vi "MeasAction.vi"(8 "error in (no error)":errorcluster caption="entrée d'erreur (pas d'erreur)", 9 "CurvePointIndex":i32, 10 "AllPointIndex":i32, 11 "InstrClassIn":refnum<class "SymphonyCCD.lvclass"> caption="DNL_LabVIEW Object in") -> (0 "error out":errorcluster caption="sortie d'erreur", 2 "MeasDatOut":dbl[](array[numeric]), 3 "InstrClassOut":refnum<class "SymphonyCCD.lvclass"> caption="DNL_LabVIEW Object out")   [LabVIEW 2019, in "SymphonyCCD.lvclass"]
uses:
  SymphonyCCD.lvclass
  SymphonyCCD.lvclass/SymphonyCCD.ctl
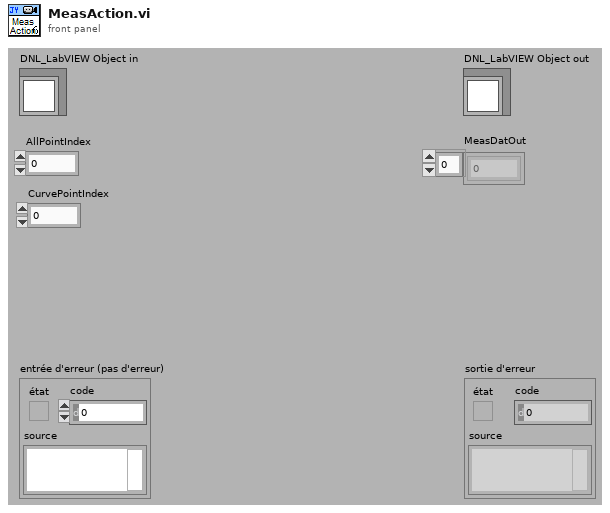
[diagram p1: front panel]
types:
  T1 = typedef "SymphonyCCD.lvclass/SymphonyCCD_Func.ctl" = enum16{"AcqImageSim (Counts)", "AcqImage (Counts)"}
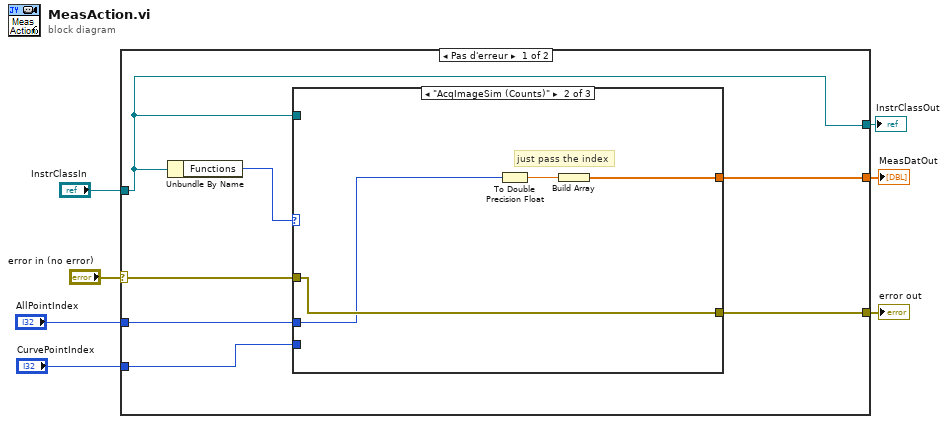
[diagram p0: block diagram]
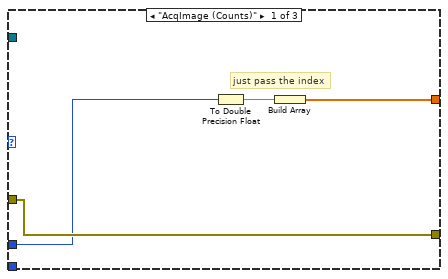
[diagram p2: hidden frame]
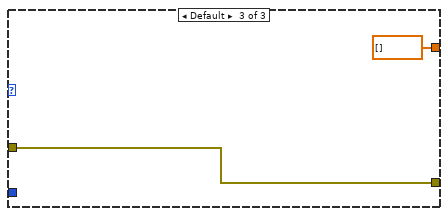
[diagram p3: hidden frame]
diagram:
  n1 = case shown="Pas d'erreur" "error in (no error)" {
    selector: "error in (no error)" -> [w10 w25]
    tunnel: "InstrClassIn" -> [w8 w26]
    tunnel: [w8 w26] -> w5
    tunnel: "AllPointIndex" -> [w14 _]
    tunnel: [w13 w25] -> w3
    tunnel: [w12 _] -> w2
    tunnel: "CurvePointIndex" -> [w9 _]
    frame No Error {
      n2 = Unbundle By Name(w8) -> ("Functions"=w11:T1)
      n3 = case shown="\"AcqImageSim (Counts)\"" w11 {
        tunnel: w14 -> [w15 w19 _]
        tunnel: [w18 w22 w23] -> w13
        tunnel: [w16 w20 dbl[] [] ("Outputs")] -> w12
        tunnel: w10 -> [w18 w22 w23]
        tunnel: w9 -> [_ _ _]
        tunnel: w8 -> [_ _ _]
        frame "AcqImage (Counts)" {
          # "just pass the index"
          n4 = To Double Precision Float(number=w15) -> (double precision float=w17:dbl)
          n5 = Build Array(w17) -> (w16:dbl[])
        }
        frame "AcqImageSim (Counts)" {
          # "just pass the index"
          n6 = To Double Precision Float(number=w19) -> (double precision float=w21:dbl)
          n7 = Build Array(w21) -> (w20:dbl[])
        }
        frame Default {
        }
      }
    }
    frame Error {
    }
  }
  "error out" <- w3
  "InstrClassOut" <- w5
  "MeasDatOut" <- w2
